vi "Global_SM_Data Out.vi"() -> ()   [LabVIEW 2017, in "Shooter.lvlib"]
uses:
  Shooter.lvlib
  Cluster_SM to HW Wheel Data.ctl
  Cluster_SM to HW Hood Data.ctl
  Cluster_SM Status.ctl
panel:
  in  "Shooter SM_Status":T1
  out "SM_Hood Data":T2
  out "SM_Wheel Data":T3
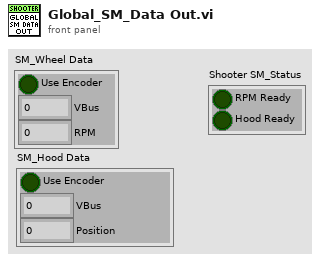
[diagram p1: front panel]
types:
  T1 = typedef "Shooter.lvlib/Cluster_SM Status.ctl" = cluster{"RPM Ready":bool, "Hood Ready":bool}
  T2 = typedef "Shooter.lvlib/Cluster_SM to HW Hood Data.ctl" = cluster{"Use Encoder":bool, "VBus":dbl, "Position":dbl}
  T3 = typedef "Shooter.lvlib/Cluster_SM to HW Wheel Data.ctl" = cluster{"Use Encoder":bool, "VBus":dbl, "RPM":dbl}
diagram:
